vi "Wait For Good Link.vi"(0 "refnum in":refnum<k20>, 7 "port":T2 items=["port 0", "port 1"], 11 "error in":errorcluster) -> (4 "refnum out":refnum<k20>, 8 "port debug info":T1, 15 "error out":errorcluster)   [LabVIEW 2020]
doc: "Waits until the link is up and running and without error.\nAfter this VI completes, the Aurora core should be fully up and running and ready to transmit and receive data.\n\n<B>Input Parameters</B>\n\n<B>Refnum in</B> Receives a reference to the FPGA from the previous VI.\n\n<B>Port</B> Specifies the port on which to check if the UserClk is running.\n\n<B>error in</B> describes error conditions that occur before this node runs. This input provides standard error in functionality.\n\n<B>Output Parameters</B>\n\n<B>Refnum out</B> passes a reference to the FPGA to the next VI.\n\n<B>Port Debug Info</B> contains debug information related to the specified Port's link status.\n\n<B>Port Debug Info.Hard Error</B> indicates whether a hard error has occurred within the Aurora core.\n\n<B>Port Debug Info.Soft Error</B> indicates whether a soft error has occurred within the Aurora core.\n\n<B>Port Debug Info.Lane Up</B> indicates whether the lanes on the specified Port are up. This contains a bitwise OR of the status of the four lanes coming from the Aurora core.\n\n<B>Port Debug Info.Channel Up</B> indicates whether the channel is up.\n\n<B>Port Debug Info.Sys Reset</B> indicates whether the Aurora core is in System reset.\n\n<B>error out</B> contains error information. This output provides standard error out functionality."
uses:
  Port.ctl
  Aurora FPGA Ref.ctl
  <vilib>/Utility/error.llb/Error Cluster From Error Code.vi
  <vilib>/rvi/errors/niLvFpgaAdjustHostInterfaceError.vi
  <vilib>/rvi/interface/nirviReadWriteControl/nirviReadWriteControl.xnode
  <vilib>/rvi/interface/Simulation/niFpgaSimulationCallBeginRW.vi
  NiFpgaLv.dll
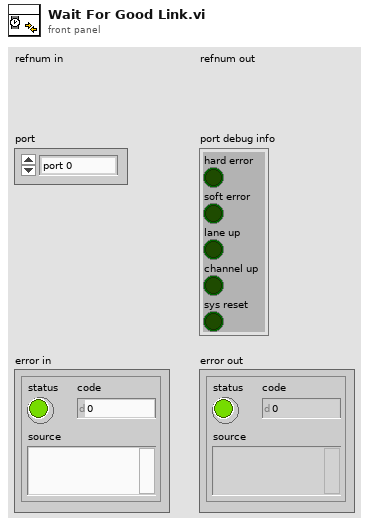
[diagram p1: front panel]
types:
  T1 = cluster{"hard error":bool, "soft error":bool, "lane up":bool, "channel up":bool, "sys reset":bool}
  T2 = typedef "Port.ctl" = i32
  T3 = typedef "Aurora FPGA Ref.ctl" = refnum<k20>
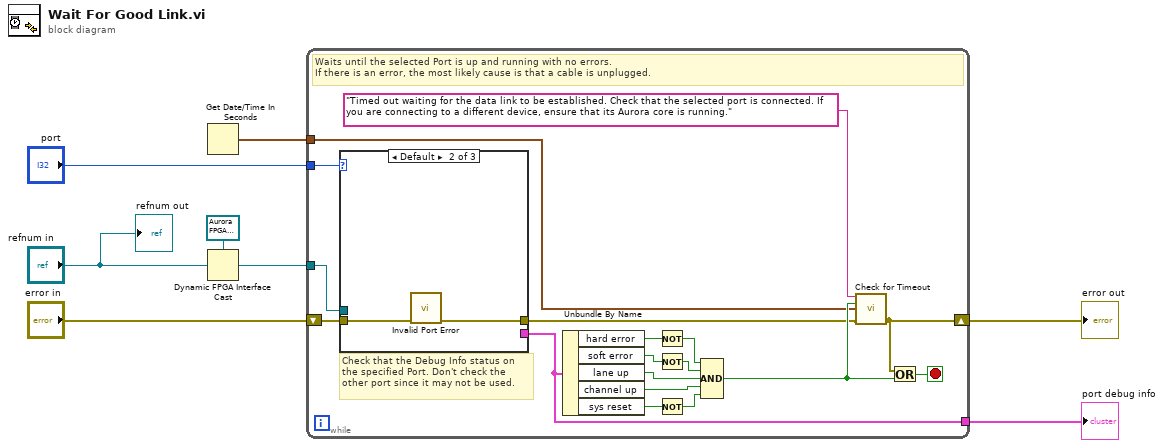
[diagram p0: block diagram]
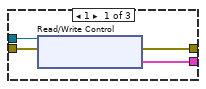
[diagram p2: hidden frame]
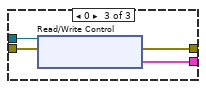
[diagram p3: hidden frame]
diagram:
  n1 = Get Date/Time In Seconds() -> (seconds since 1Jan1904=w8:timestamp)
  n2 = Dynamic FPGA Interface Cast(Session In=T3 refnum ("USRP RIO Streaming Xcvr FPGA VI Reference"), Type="refnum in") -> (Session Out=w6:T3)
  n3 = while {
    shift-right: [w12] -> w3
    shift-left: "error in" -> [w24]
    tunnel: w8 -> [w10]
    tunnel: [w23] -> w2
    tunnel: w6 -> [w25]
    tunnel: "port" -> [w9]
    stop <- w26 stop-if-true
    # "Check that the Debug Info status on\nthe specified Port. Don't check the \nother port since it may not be used."
    # "Waits until the selected Port is up and running with no errors.\nIf there is an error, the most likely cause is that a cable is unplugged."
    n4 = case shown="Default" w9 {
      tunnel: w25 -> [w30 _ w36]
      tunnel: w24 -> [w29 w31 w35]
      tunnel: [w28 w32 w34] -> w11
      tunnel: [w27 _ w33] -> w23
      frame 1 {
        n5 = xnode "Read/Write Control"("FPGA VI Reference In"=w30, "error in"=w29) -> ("error out"=w28:errorcluster, "sfp 1.debug info"=w27:T1)  [unwired: 1 out]
      }
      frame Default {
        n6 = call "Invalid Port Error.vi"("error in"=w31) -> ("error out"=w32:errorcluster)  [unwired: 14 in]
      }
      frame 0 {
        n7 = xnode "Read/Write Control"("FPGA VI Reference In"=w36, "error in"=w35) -> ("error out"=w34:errorcluster, "sfp 0.debug info"=w33:T1)  [unwired: 1 out]
      }
    }
    n8 = Unbundle By Name(w23) -> ("hard error"=w22:bool, "soft error"=w21:bool, "lane up"=w20:bool, "channel up"=w19:bool, "sys reset"=w18:bool)
    n9 = Not(x=w22) -> (.not. x?=w16:bool)
    n10 = Not(x=w21) -> (.not. x?=w17:bool)
    n11 = Not(x=w18) -> (.not. x?=w15:bool)
    n12 = Compound Arithmetic op=AND(w16, w17, w20, w19, w15) -> (w13:bool)
    n13 = call "Check for Timeout.vi"("error message"="Timed out waiting for the data link to be established. Check that the selected port is connected. If you are connecting to a different device, ensure that its Aurora core is running." ("error message (\"\")"), "complete?"=w13, "start time"=w10, "error in"=w11) -> ("error out"=w12:errorcluster)  [unwired: 11 in]
    n14 = Or(x=w12, y=w13) -> (x .or. y?=w26:bool)
  }
  "error out" <- w3
  "port debug info" <- w2
  "refnum out" <- "refnum in"
